vi "get mapped action channels.vi"(7 "owner":string, 11 "sequencer configuration in":refnum<class "base TBM sequencer configuration.lvclass">) -> (2 "action channels":refnum<class "TBM channel.lvclass">[](array[class]), 3 "sequencer configuration out":refnum<class "base TBM sequencer configuration.lvclass">)   [LabVIEW 2014, in "base TBM sequencer configuration.lvclass"]
uses:
  base TBM sequencer configuration.lvclass
  <vilib>/NI/Tag Bus Module Framework/channel/TBM channel.lvclass
  <vilib>/NI/Tag Bus Module Framework/channel/channel classification.ctl
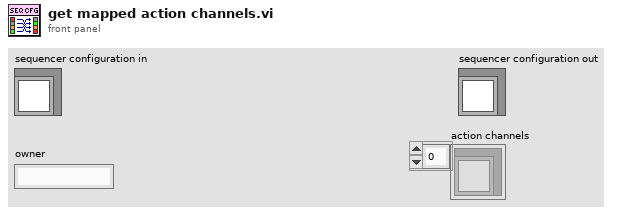
[diagram p1: front panel]
types:
  T1 = typedef "TBM channel.lvclass/channel classification.ctl" = enum16{"input data", "output data", "processing parameter", "processing result"}
  T2 = typedef "base TBM sequencer configuration.lvclass/Module Mappings.ctl" = cluster{"Owning ID":string, "Input Mappings":T3[], "Process Parameter Mappings":T3[], "Process Results Mappings":T3[], "Output Mappings":T3[]}
  T3 = typedef "tag bus.lvlib/data table.lvlib/mapping specification.ctl" = cluster{"data type":T4, "mappings":T5[]}
  T4 = typedef "tag bus.lvlib/tag descriptor.lvclass/Data Type.ctl" = enum16{"Double", "Single", "I64", "I32", "I16", "I8", "U64", "U32", "U16", "U8", "Boolean", "String", "Array of Double", "Array of Single", "Array of I64", "Array of I32", "Array of I16", "Array of I8", "Array of U64", "Array of U32", "Array of U16", "Array of U8", "Array of Boolean", "Array of String"}
  T5 = typedef "tag bus.lvlib/data table.lvlib/mapping.ctl" = cluster{"sink name":string, "source name":string}
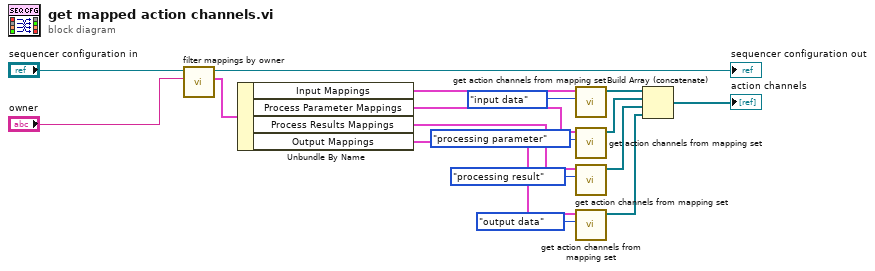
[diagram p0: block diagram]
diagram:
  n1 = call "filter mappings by owner.vi"("owner"="owner", "engine configuration in"="sequencer configuration in") -> ("module mapping"=w14:T2, "engine configuration out"=→"sequencer configuration out":refnum<class "base TBM sequencer configuration.lvclass">)  [unwired: 8 in]
  n2 = Unbundle By Name(w14) -> ("Input Mappings"=w13:T3[], "Process Parameter Mappings"=w11:T3[], "Process Results Mappings"=w10:T3[], "Output Mappings"=w9:T3[])
  n3 = call "get action channels from mapping set.vi"("channel classification"=channel_classification."input data", "mappings set"=w13) -> ("action channels"=w5:refnum<class "TBM channel.lvclass">[])  [unwired: 9 in]
  n4 = call "get action channels from mapping set.vi"("channel classification"=channel_classification."processing parameter", "mappings set"=w11) -> ("action channels"=w4:refnum<class "TBM channel.lvclass">[])  [unwired: 9 in]
  n5 = call "get action channels from mapping set.vi"("channel classification"=channel_classification."processing result", "mappings set"=w10) -> ("action channels"=w3:refnum<class "TBM channel.lvclass">[])  [unwired: 9 in]
  n6 = call "get action channels from mapping set.vi"("channel classification"=channel_classification."output data", "mappings set"=w9) -> ("action channels"=w2:refnum<class "TBM channel.lvclass">[])  [unwired: 9 in]
  n7 = Build Array (concatenate)(w5, w4, w3, w2) -> (→"action channels":refnum<class "TBM channel.lvclass">[])
